vi "Natural Logarithm.vi"   [LabVIEW 2017, in "NI_Matrix.lvlib"]
doc: "Computes the natural logarithm of the input matrix."
uses:
  <vilib>/Analysis/Matrix/NI_Matrix.lvlib
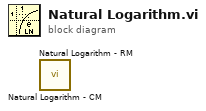
[diagram p0: block diagram]
diagram:
  n1 = call <vilib>:"Natural Logarithm - CM.vi"() -> ()  [unwired: 1 in, 1 out]
  n2 = call <vilib>:"Natural Logarithm - RM.vi"() -> ()  [unwired: 1 in, 1 out]
